vi "cursor_move.vi"(7 "xy_graph_reference":refnum<vi>, 8 "error in (no error)":errorcluster, 10 "cursor_index":i32, 11 "active_cursor":u32) -> (0 "error out":errorcluster)   [LabVIEW 2015, in "lv-graph.lvlib"]
doc: "This VI provides the ability to move an active cursor (providing the X and Y values) indexed by the active cursor input."
uses:
  lv-graph.lvlib
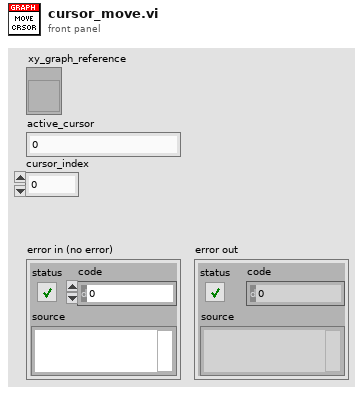
[diagram p1: front panel]
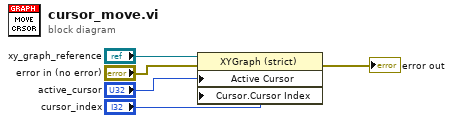
[diagram p0: block diagram]
diagram:
  n1 = property class="XYGraph (strict)"(reference="xy_graph_reference", error in="error in (no error)", "Active Cursor"="active_cursor", "Cursor.Cursor Index"="cursor_index") -> (error out=→"error out":errorcluster)  [unwired: 1 out]
